vi "esp32_blink.vi"() -> ()   [LabVIEW 2025]
uses:
  <vilib>/Instr/_visa.llb/VISA Configure Serial Port (Instr).vi
panel:
  in  "Serial Port":refnum<visa-resource-name>="COM1"
  in  "End Program":bool
  out "LED State":bool
  in  "LED Toggle":bool
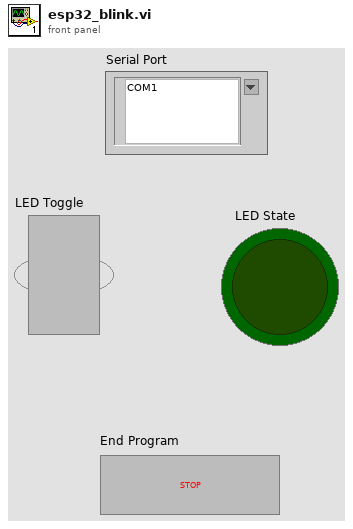
[diagram p1: front panel]
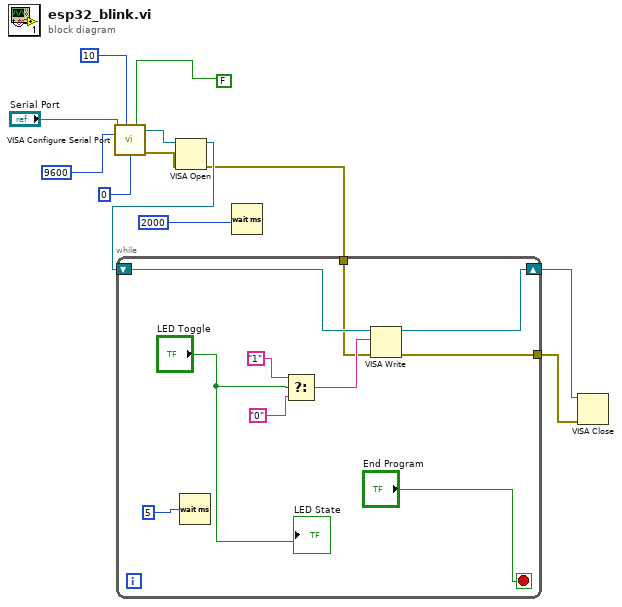
[diagram p0: block diagram]
diagram:
  n1 = call-poly "VISA Configure Serial Port"("VISA resource name"="Serial Port", "timeout (10sec)"=10, "Enable Termination\nChar (T)"=FALSE ("Enable Termination\nChar (T)"), "baud rate (9600)"=9600, "flow control (0:none)"=0) -> ("VISA resource name out"=w11:refnum<visa-resource-name>, "error out"=w3:errorcluster)  [unwired: 9 in]
  n2 = VISA Open(error in (no error)=w3, VISA resource name=w11) -> (VISA resource name=w12:refnum<visa-resource-name>, error out=w5:errorcluster)  [unwired: 3 in]
  n3 = while {
    tunnel: [w18] -> w6
    tunnel: w5 -> [w13]
    shift-right: [w19] -> w7
    shift-left: w12 -> [w20]
    stop <- "End Program" stop-if-true
    n4 = Wait (ms)(milliseconds to wait=5) -> ()  [unwired: 1 out]
    n5 = Select(t="1", s="LED Toggle", f="0") -> (s? t:f=w17:string)
    n6 = VISA Write(VISA resource name=w20, write buffer=w17, error in (no error)=w13) -> (VISA resource name out=w19:refnum<visa-resource-name>, error out=w18:errorcluster)  [unwired: 1 out]
    "LED State" <- "LED Toggle"
  }
  n7 = Wait (ms)(milliseconds to wait=2000) -> ()  [unwired: 1 out]
  n8 = VISA Close(VISA resource name=w7, error in (no error)=w6) -> ()  [unwired: 1 out]
